vi "Init Google OAuth.vi"(5 "Required Scope(s) (gmail.send)":string[](array[string])=["https://www.googleapis.com/auth/gmail.send"], 7 "Redirect URL (http://localhost)":string, 8 "error in (no error)":errorcluster, 10 "OAuth2:Client":refnum<class "Client.lvclass">, 11 "Account (Prompt)":string) -> (0 "error out":errorcluster, 3 "Google out":refnum<class "Google.lvclass">)   [LabVIEW 2020, in "OAuth2.lvlib" / "Google.lvclass"]
doc: "Initializes a Google authorization provider instance. The class inherits from OAuth2:OAuth2 and once the instance is created, Do Auth.vi or Refresh Auth.vi can be called.\n\nThis VI defaults to requesting authorization to send emails on behalf of an account but the Scopes can be customized to other Google API scopes as necessary. If known, the user's Google account can be specified otherwise the user will select which account to authorize access to during authorization."
uses:
  Google.lvclass
  OAuth2/OAuth2.lvclass
  Request/Request.lvclass
  Client/Client.lvclass
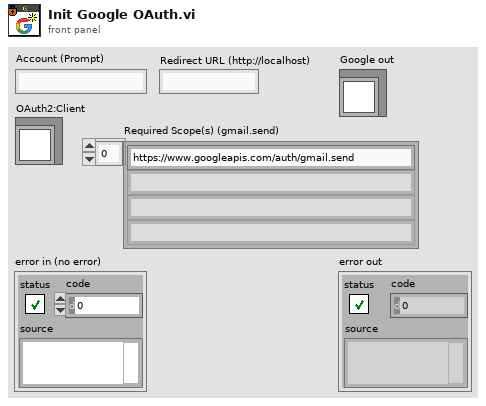
[diagram p1: front panel]
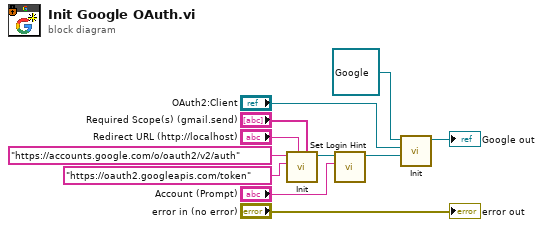
[diagram p0: block diagram]
diagram:
  n1 = call "Init.vi"("Required Scope(s)"="Required Scope(s) (gmail.send)", "Redirect URL (http://localhost)"="Redirect URL (http://localhost)", "Token URL"="https://oauth2.googleapis.com/token" ("url"), "Auth URL"="https://accounts.google.com/o/oauth2/v2/auth" ("url")) -> ("Request out"=w5:refnum<class "Request.lvclass">)  [unwired: 7 in]
  n2 = call "Set Login Hint.vi"("Login Hint"="Account (Prompt)", "Request in"=w5) -> ("Request out"=w3:refnum<class "Request.lvclass">)  [unwired: 9 in]
  n3 = call "Init.vi"("Request"=w3, "Client"="OAuth2:Client", "OAuth2 in (New)"=refnum<class "Google.lvclass"> refnum ("Google in")) -> ("OAuth2"=→"Google out":refnum<class "Google.lvclass">)  [unwired: 8 in]
  "error out" <- "error in (no error)"
